vi "SetIMOrder.vi"(6 "Legacy (f)?":bool, 8 "error in (no error)":errorcluster, 10 "IMOrder":u8) -> (0 "error out":errorcluster)   [LabVIEW 2011]
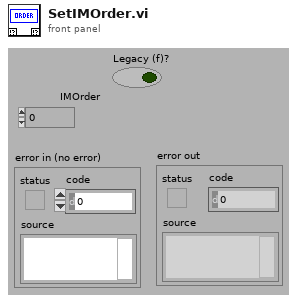
[diagram p1: front panel]
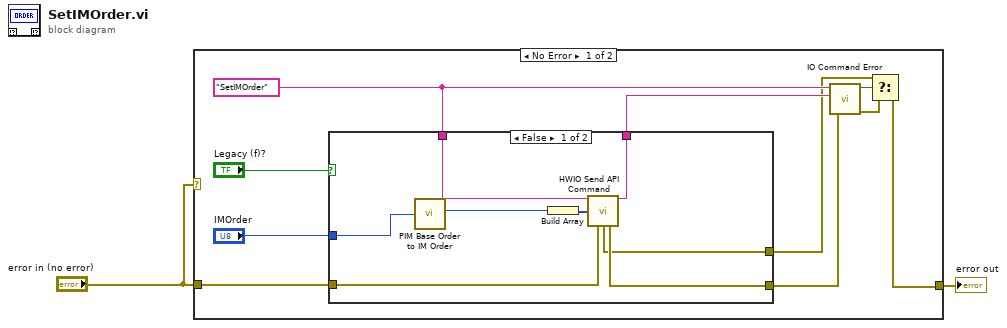
[diagram p0: block diagram]
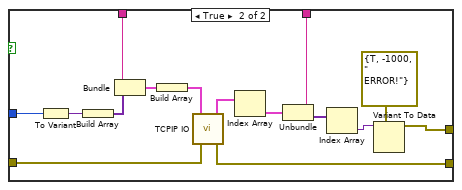
[diagram p2: hidden frame]
diagram:
  n1 = case shown="No Error" "error in (no error)" {
    tunnel: "error in (no error)" -> [w11 w36]
    tunnel: [w4 w36] -> w2
    frame No Error {
      w9 = "SetIMOrder"
      n2 = case shown="False" "Legacy (f)?" {
        tunnel: "IMOrder" -> [w14 w35]
        tunnel: w11 -> [w20 w32]
        tunnel: [w19 w30] -> w10
        tunnel: w9 -> [w17 w29]
        tunnel: [w18 w25] -> w8
        tunnel: [w15 w21] -> w5
        frame False {
          n3 = call "PIM Base Order to IM Order.vi"("Base Order (0)"=w14) -> ("IM Order"=w13:u8)  [unwired: 4 in, 1 out]
          n4 = Build Array(w13) -> (w16:u8[])
          n5 = call "HWIO Send API Command.vi"("Action"=w17, "Integer"=w16, "error in (no error)"=w20) -> ("Action out"=w18:string, "HWError"=w15:errorcluster, "error out"=w19:errorcluster)  [unwired: 5 in, 5 out]
        }
        frame True {
          n6 = To Variant(anything=w35) -> (Variant=w34:variant)
          n7 = Build Array(w34) -> (w33:variant[])
          n8 = Bundle(w29, w33) -> (w31:cluster{string, variant[]})  [unwired: 1 out]
          n9 = Build Array(w31) -> (w28:cluster{string, variant[]}[])
          n10 = call "TCPIP IO.vi"("error in (no error)"=w32, "Commands"=w28) -> ("error out"=w30:errorcluster, "Responses"=w26:cluster{string, variant[]}[])  [unwired: 1 in, 3 out]
          n11 = Index Array(array=w26) -> (element=w27:cluster{string, variant[]})  [unwired: 1 in]
          n12 = Unbundle(w27) -> (w25:string, w22:variant[])
          n13 = Index Array(array=w22) -> (element=w24:variant)  [unwired: 1 in]
          n14 = Variant To Data(type=errorcluster {"status"=TRUE, "code"=-1000, "source"=" ERROR!"} ("error out"), Variant=w24) -> (data=w21:errorcluster)  [unwired: 1 in, 1 out]
        }
      }
      n15 = call "IO Command Error.vi"("error in (no error)"=w10, "Command Returned (\"\")"=w8, "Command Sent (\"\")"=w9) -> ("error out"=w6:errorcluster, "HW ERR?"=w7:bool)  [unwired: 3 out]
      n16 = Select(t=w5, s=w7, f=w6) -> (s? t:f=w4:errorcluster)
    }
    frame Error {
    }
  }
  "error out" <- w2
